vi "Date String To Time Stamp.vi"(7 "error in (no error)":errorcluster, 11 "Date":string) -> (3 "Time Stamp":timestamp, 5 "error out":errorcluster)   [LabVIEW 2017, in "Feed.lvclass"]
uses:
  <vilib>/NI_RSS/Feed/Feed.lvclass
  <vilib>/Utility/miscctls.llb/LVDateTimeRec.ctl
panel:
  # "2008-09-25T13:57:00Z"
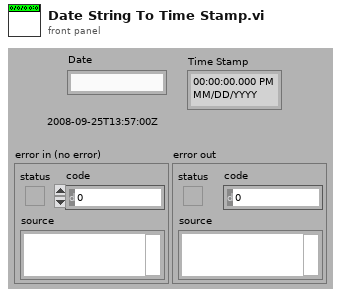
[diagram p1: front panel]
types:
  T1 = typedef "LVDateTimeRec.ctl" = cluster{"fractional second":dbl, "second":i32, "minute":i32, "hour":i32, "day of month":i32, "month":i32, "year":i32, "day of week":i32, "day of year":i32, "DST":i32}
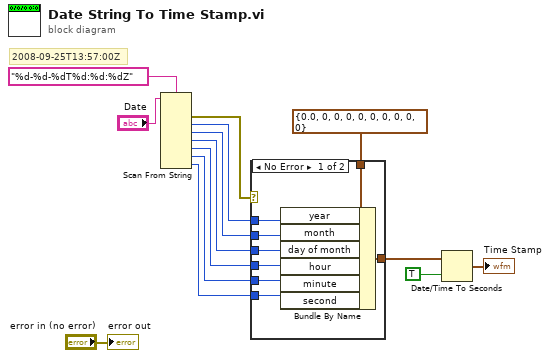
[diagram p0: block diagram]
diagram:
  # "2008-09-25T13:57:00Z"
  n1 = Scan From String(format string="%d-%d-%dT%d:%d:%dZ", input string="Date") -> (error out=w1:errorcluster, output 1=w12:i32, output 2=w10:i32, output 3=w9:i32, output 4=w8:i32, output 5=w7:i32, output 6=w6:i32)  [unwired: 8 in, 2 out]
  n2 = case shown="No Error" w1 {
    tunnel: w12 -> [w22 _]
    tunnel: T1 {"fractional second"=0.0, "second"=0, "minute"=0, "hour"=0, "day of month"=0, "month"=0, "year"=0, "day of week"=0, "day of year"=0, "DST"=0} ("date time rec") -> [w21 w23]
    tunnel: w10 -> [w20 _]
    tunnel: w9 -> [w19 _]
    tunnel: w8 -> [w18 _]
    tunnel: w7 -> [w17 _]
    tunnel: w6 -> [w16 _]
    tunnel: [w15 w23] -> w4
    frame No Error {
      n3 = Bundle By Name(cluster=w21, "year"=w22, "month"=w20, "day of month"=w19, "hour"=w18, "minute"=w17, "second"=w16) -> (w15:T1)
    }
    frame Error {
    }
  }
  n4 = Date/Time To Seconds(1:TRUE ("is UTC (F)"), 2:w4) -> (0:→"Time Stamp":timestamp)
  "error out" <- "error in (no error)"
